vi "XML Build Poll Range.vi"(2 "XML-Message alt":string, 3 "von EVID-Nr":i32, 8 "bis EVID-Nr":i32) -> (0 "Attribut Name (Range)":string, 5 "Anzahl Elemente":i32, 7 "XML-Message neu":string)   [LabVIEW 2020, in "FT-IR.lvlib" / "TOOLweb Interface.lvlib" / "TOOLweb Interface Hilfs-VIs.lvlib"]
doc: "Fügt an die bisher aufgebauten XML-Poll-Request-Zeilen \"XML-Message alt\" eine Poll-Request-Zeile hinzu, die alle Variablen im Bereich von \"von EVID-Nr\" bis \"bis EVID-Nr\" anfordert.\n\nDie Ausgänge \"Attribut Name (Range)\" und \"Anzahl Elemente\" werden zu einem auf gleicher Höhe liegendem XML-Parser verbunden, der damit keine weiteren Informationen benötigt.\n\nDer Ausgangs-String \"XML-Message neu\" wird an ein weiteres XML-Build-VI oder an das abschließende \"XML Build Poll Request Frame\" übergeben, das allen Zeilen gemeinsam mit dem Start-Tag <PollRequest> und dem End-Tag </PollRequest> den Rahmen für eine einzige und damit schnelle XML-Anfrage gibt."
uses:
  TOOLweb Interface Hilfs-VIs.lvlib
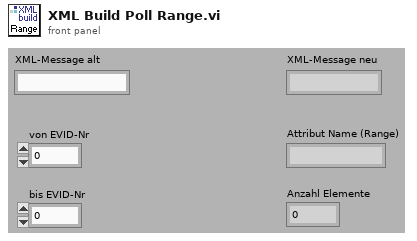
[diagram p1: front panel]
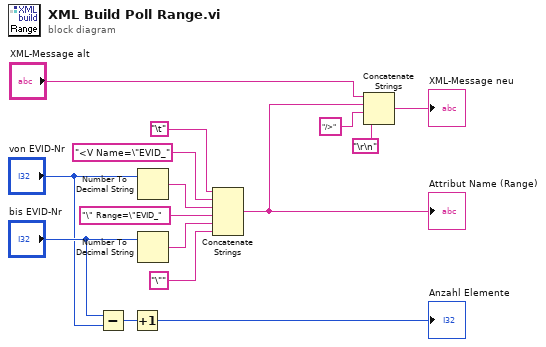
[diagram p0: block diagram]
diagram:
  n1 = Subtract(x="bis EVID-Nr", y="von EVID-Nr") -> (x-y=w2:i32)
  n2 = Increment(x=w2) -> (x+1=→"Anzahl Elemente":i32)
  n3 = Number To Decimal String(number="von EVID-Nr") -> (decimal integer string=w13:string)  [unwired: 1 out]
  n4 = Number To Decimal String(number="bis EVID-Nr") -> (decimal integer string=w12:string)  [unwired: 1 out]
  n5 = Concatenate Strings("\t", "<V Name=\"EVID_" ("Daten (Eingang)"), w13, "\" Range=\"EVID_" ("Daten (Eingang)"), w12, "\"" ("Daten (Eingang)")) -> (w8:string)
  "Attribut Name (Range)" <- w8
  n6 = Concatenate Strings("XML-Message alt", w8, "/>" ("Daten (Eingang)"), "\r\n") -> (→"XML-Message neu":string)
